vi "wait.vi"(7 "waitgroup":T1, 8 "error in (no error)":errorcluster, 10 "skip_done":bool, 11 "wait_ms":u32) -> (0 "error out":errorcluster)   [LabVIEW 2015, in "lv-waitgroup.lvlib"]
uses:
  lv-waitgroup.lvlib
  public/_controls/api_waitgroup.ctl
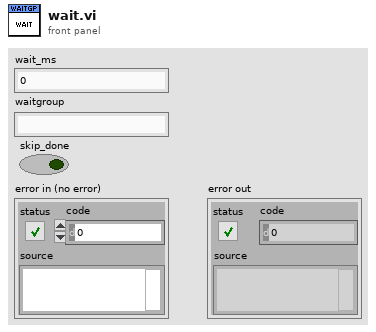
[diagram p1: front panel]
types:
  T1 = typedef "lv-waitgroup.lvlib/api_waitgroup.ctl" = string
  T2 = typedef "lv-waitgroup.lvlib/api_child_queue.ctl" = string
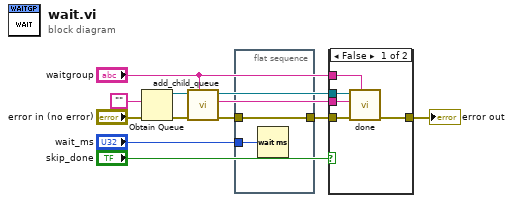
[diagram p0: block diagram]
diagram:
  n1 = Obtain Queue(element data type="", error in (no error)="error in (no error)") -> (queue out=w2:refnum<queue>, error out=w7:errorcluster)  [unwired: 3 in, 1 out]
  n2 = call "add_child_queue.vi"("waitgroup"="waitgroup", "error in (no error)"=w7, "queue"=w2) -> ("error out"=w9:errorcluster, "child_id"=w1:T2)  [unwired: 7 in]
  n3 = flat-sequence {
    tunnel: "wait_ms" -> [w13]
    tunnel: w9 -> [w12]
    tunnel: [w12] -> w6
    frame #0 {
      n4 = Wait (ms)(milliseconds to wait=w13) -> ()  [unwired: 1 out]
    }
  }
  n5 = case shown="False" "skip_done" {
    tunnel: [w18 w19] -> w10
    tunnel: "waitgroup" -> [w17 _]
    tunnel: w6 -> [w16 w19]
    tunnel: w2 -> [w15 _]
    tunnel: w1 -> [w14 _]
    frame False {
      n6 = call "done.vi"("waitgroup"=w17, "error in (no error)"=w16, "child_id"=w14, "queue"=w15) -> ("error out"=w18:errorcluster)  [unwired: 7 in]
    }
    frame True {
    }
  }
  "error out" <- w10
